vi "image global.vi"() -> ()   [LabVIEW 2013]
panel:
  out "valveV2":picture
  out "valveV1":picture
  out "PIPE3 90":picture
  out "PIPE2 90":picture
  out "PIPE1 90":picture
  out "PIPE0 90":picture
  out "UND6 3":picture
  out "UND6 2":picture
  out "UND6 1":picture
  out "UND5 3":picture
  out "UND5 2":picture
  out "UND5 1":picture
  out "UND4 3":picture
  out "UND4 2":picture
  out "UND4 1":picture
  out "UND6 0":picture
  out "UND5 0":picture
  out "UND4 0":picture
  out "SAC3 3":picture
  out "SAC3 2":picture
  out "SAC3 1":picture
  out "SAC3 0":picture
  out "SAC2 3":picture
  out "SAC2 2":picture
  out "SAC2 1":picture
  out "SAC2 0":picture
  out "SACPIPE2 2":picture
  out "SACPIPE2 1":picture
  out "SACPIPE2 0":picture
  out "SACPIPE1 2":picture
  out "SACPIPE1 1":picture
  out "SACPIPE1 0":picture
  out "UPIPE2 2":picture
  out "UPIPE2 1":picture
  out "UPIPE2 0":picture
  out "UPIPE1 2":picture
  out "UPIPE1 1":picture
  out "UPIPE1 0":picture
  out "PPIPE 2":picture
  out "PPIPE 1":picture
  out "PPIPE 0":picture
  out "HPIPE270 2":picture
  out "HPIPE270 1":picture
  out "HPIPE270 0":picture
  out "HPIPE180 2":picture
  out "HPIPE180 1":picture
  out "HPIPE180 0":picture
  out "HPIPE90 2":picture
  out "HPIPE90 1":picture
  out "HPIPE90 0":picture
  out "HPIPE0 2":picture
  out "HPIPE0 1":picture
  out "HPIPE0 0":picture
  out "ROUGHMAN2":picture
  out "ROUGHMAN1":picture
  out "ROUGHMAN0":picture
  out "BACKMAN2":picture
  out "BACKMAN 1":picture
  out "BACKMAN 0":picture
  out "EPX FAULT":picture
  out "UND3 3":picture
  out "UND3 2":picture
  out "UND3 1":picture
  out "UND2 3":picture
  out "UND2 2":picture
  out "UND2 1":picture
  out "UND1 3":picture
  out "UND1 2":picture
  out "UND1 1":picture
  out "UND3 0":picture
  out "UND2 0":picture
  out "UND1 0":picture
  out "SAC1 3":picture
  out "SAC1 2":picture
  out "SAC1 1":picture
  out "SAC1 0":picture
  out "PIPE3":picture
  out "PIPE2":picture
  out "PIPE1":picture
  out "PIPE0":picture
  out "Turbo 270P":picture
  out "Turbo 270 Fault":picture
  out "Turbo 270 On":picture
  out "Turbo 270R":picture
  out "Turbo 270 Off":picture
  out "Turbo 90P":picture
  out "Turbo 90 Fault":picture
  out "Turbo 90 On":picture
  out "Turbo 90R":picture
  out "Turbo 90 Off":picture
  out "Turbo 0P":picture
  out "Turbo 0 Fault":picture
  out "Turbo 0 On":picture
  out "Turbo 0R":picture
  out "Turbo 0 Off":picture
  out "EPX OFF":picture
  out "EPX ON":picture
  out "EPX P":picture
  out "EPX R":picture
  out "valveVP":picture
  out "valveVR":picture
  out "valveV0":picture
  out "valveHP":picture
  out "valveHR":picture
  out "valveH2":picture
  out "valveH1":picture
  out "valveH0":picture
  out "smallvalveP":picture
  out "smallvalveR":picture
  out "smallvalve2":picture
  out "smallvalve1":picture
  out "smallvalve0":picture
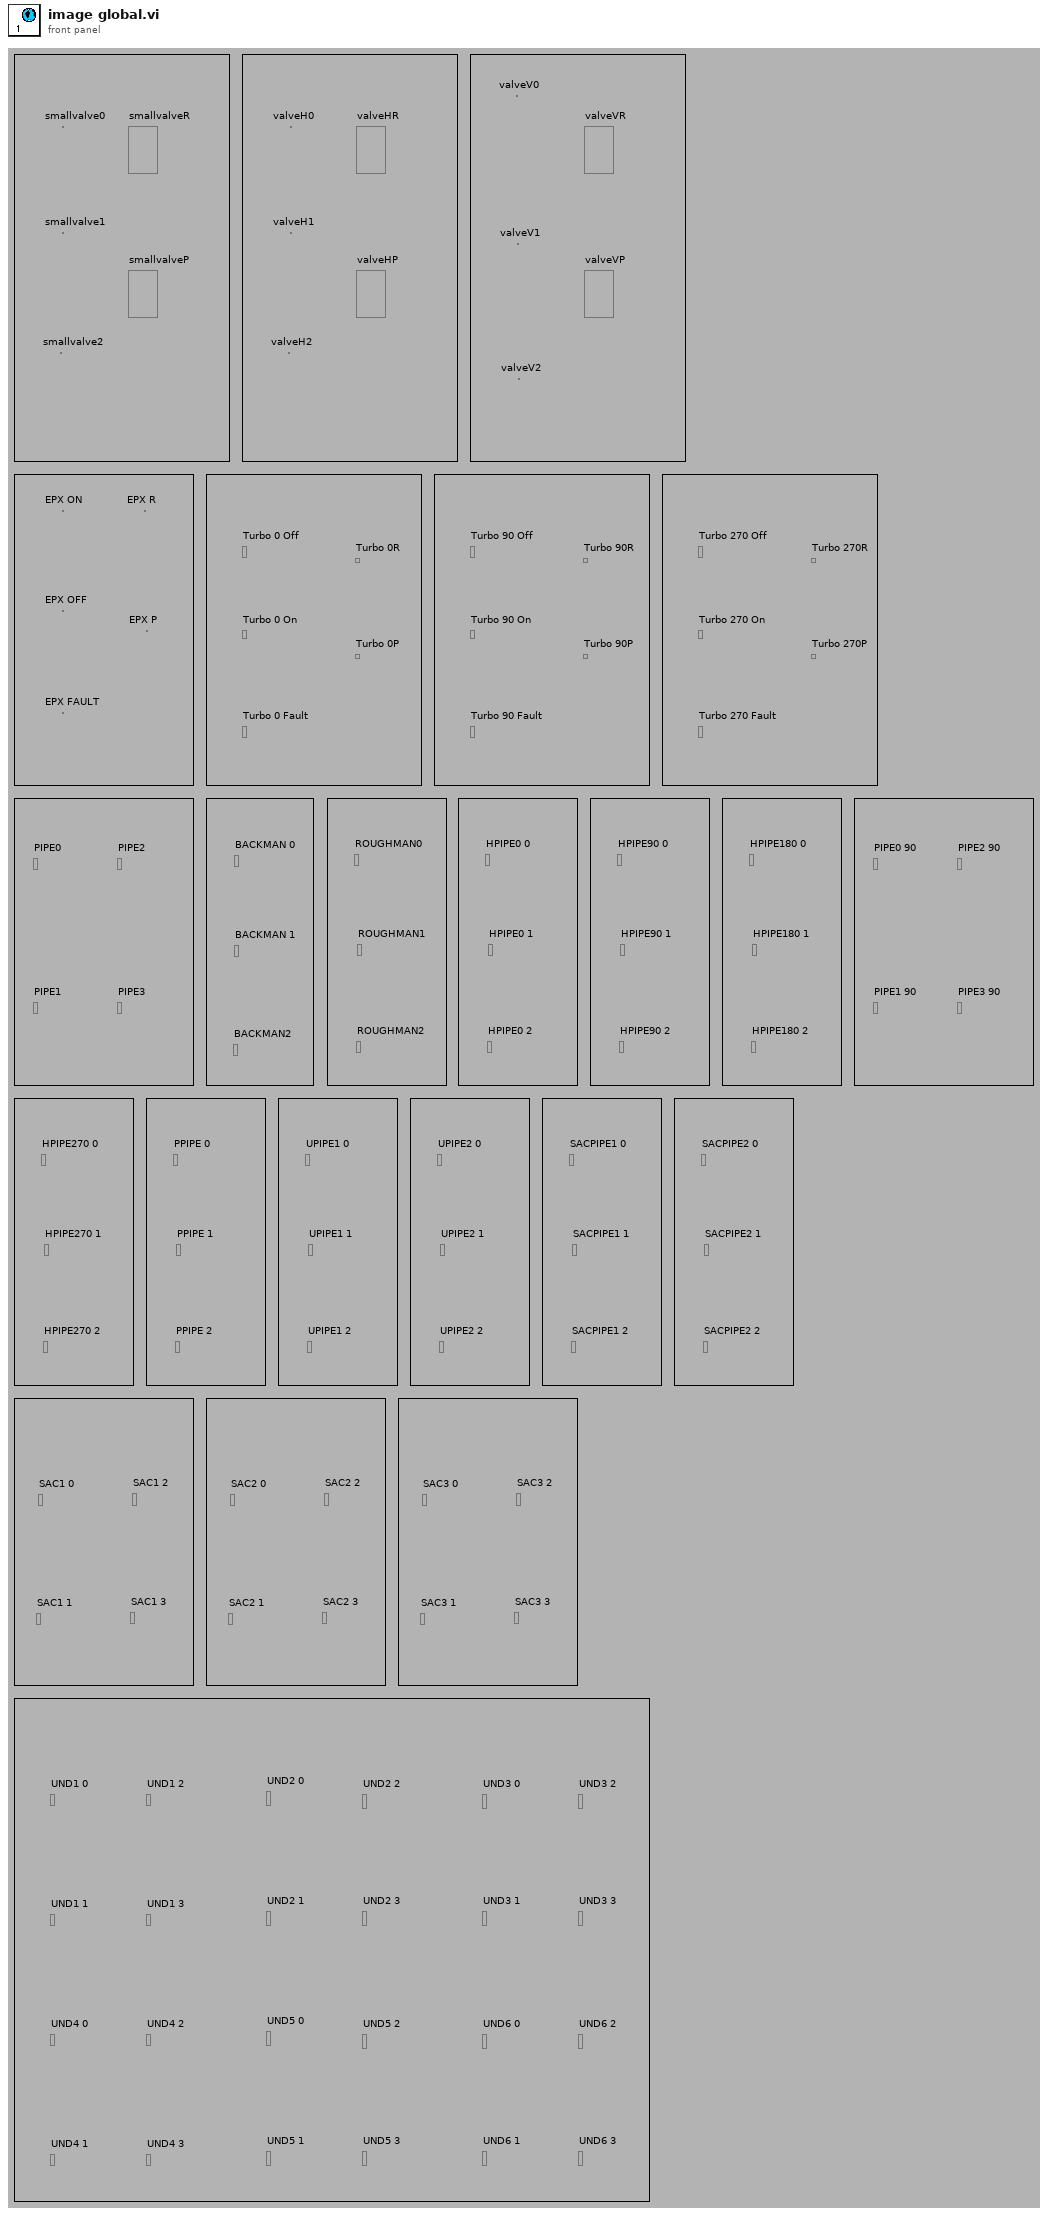
[diagram p1: front panel]
diagram:
